vi "Part 2.vi"(11 "Input":string) -> (3 "Output":i64)   [LabVIEW 2021]
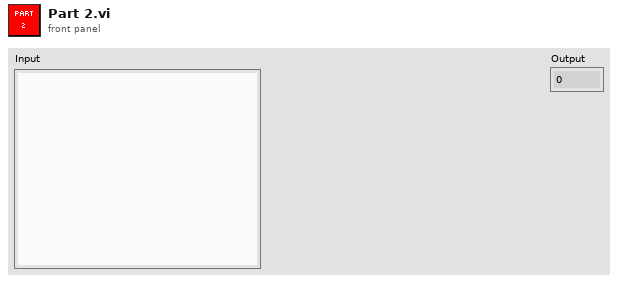
[diagram p1: front panel]
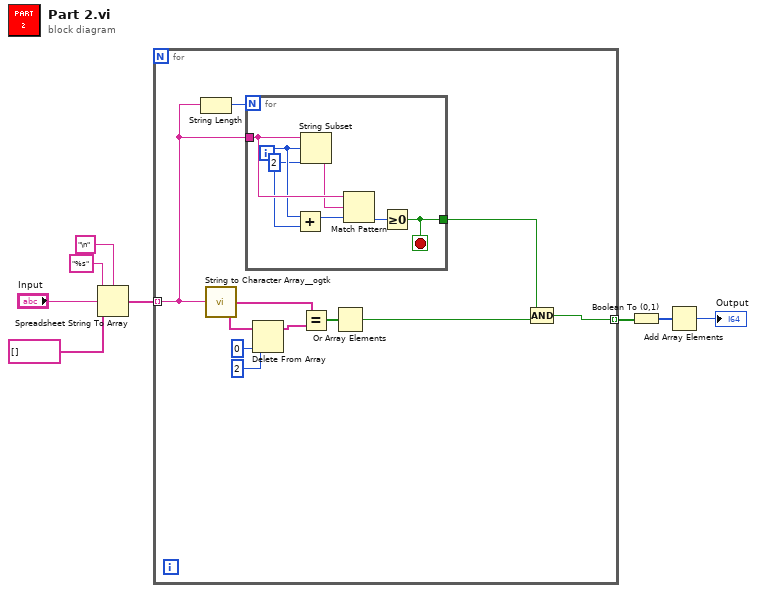
[diagram p0: block diagram]
diagram:
  n1 = Spreadsheet String To Array(delimiter (Tab)="\n", format string="%s", spreadsheet string="Input", array type (2D Dbl)=string[] []) -> (array=w4:string[])
  n2 = for {
    tunnel: w4 -> [w10] mode=indexing
    tunnel: [w12] -> w2 mode=indexing
    n3 = String Length(string=w10) -> (length=w11:i32)
    n4 = call <userlib>:"String to Character Array__ogtk.vi"("Input String"=w10) -> ("Character Array"=w15:string[])
    n5 = for {
      N: w11 -> [_]
      tunnel: w10 -> [w25]
      tunnel: [w19] -> w9
      i -> [w22]
      stop <- w19 stop-if-true
      w21 = 2 ("length (rest)")
      n6 = Add(x=w22, y=w21) -> (x+y=w23:i32)
      n7 = String Subset(string=w25, offset (0)=w22, length (rest)=w21) -> (substring=w24:string)
      n8 = Match Pattern(string=w25, regular expression=w24, offset (0)=w23) -> (offset past match=w20:i32)  [unwired: 3 out]
      n9 = Greater Or Equal To 0?(x=w20) -> (x >= 0?=w19:bool)
    }
    n10 = Delete From Array(array=w15, length=2, index=0) -> (array with subset deleted=w16:string[])  [unwired: 1 out]
    n11 = Equal?(x=w15, y=w16) -> (x = y?=w14:bool[])
    n12 = Or Array Elements(Boolean array=w14) -> (logical OR=w13:bool)
    n13 = Compound Arithmetic op=AND(w9, w13) -> (w12:bool)
  }
  n14 = Boolean To (0,1)(Boolean=w2) -> (0, 1=w3:i16[])
  n15 = Add Array Elements(numeric array=w3) -> (sum=→"Output":i16)
